vi "io_clear_buffers.vi"(6 "Block Logging (F)":bool, 8 "error in":errorcluster, 11 "VISA resource name":refnum<visa-resource-name>) -> (0 "error out":errorcluster, 3 "VISA resource name out":refnum<visa-resource-name>)   [LabVIEW 2014, in "rszvl_rsidr_core.lvlib"]
uses:
  rszvl_rsidr_core.lvlib
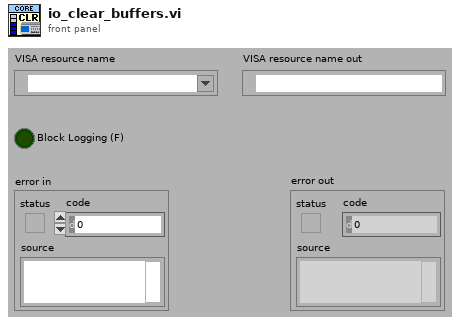
[diagram p1: front panel]
types:
  T1 = typedef "rszvl_rsidr_core.lvlib/type_Session_Data.ctl" = cluster{"Instr type":string, "Instr type for err. msg.":string, "Installed Options":string[], "OPC Timeout":i32, "Query Instrument Status":bool, "Check Range":bool, "Check Options":bool, "Add LF to Write":bool, "Simulate":bool, "Logging":bool, "Logging params":variant, "Interface Type":enum16{"Unknown", "GPIB", "VXI", "GPIB_VXI", "ASRL", "PXI", "TCPIP", "USB", "SOCKET"}, "Fast Sweep":i32, "AdditionalFlags":i32, "WaitBeforeWrite":i32, "WaitBeforeRead":i32, "BinDataChunkSize":i64}
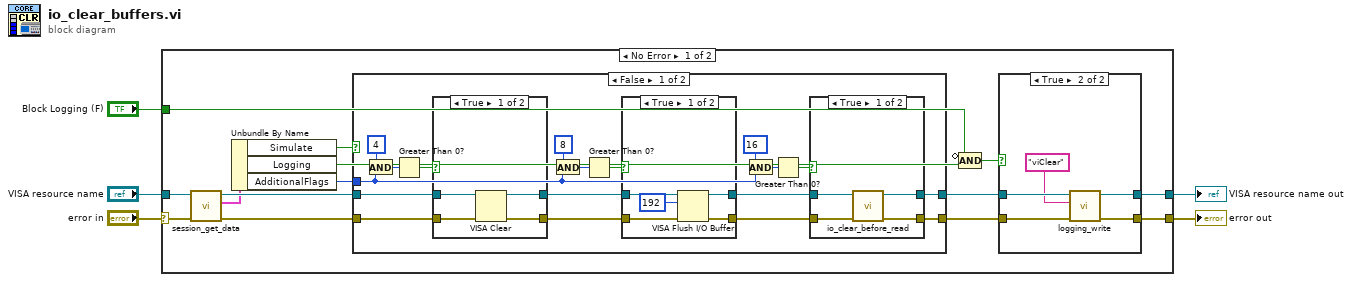
[diagram p0: block diagram]
diagram:
  n1 = case shown="No Error" "error in" {
    selector: "error in" -> [w19 w67]
    tunnel: [w13 w67] -> w1
    tunnel: "VISA resource name" -> [w18 w66]
    tunnel: [w10 w66] -> w2
    tunnel: "Block Logging (F)" -> [w6 _]
    frame No Error {
      n2 = call "session_get_data.vi"("error in"=w19, "VISA resource name"=w18) -> ("error out"=w17:errorcluster, "Session User Data out"=w15:T1, "VISA resource name out"=w16:refnum<visa-resource-name>)  [unwired: 7 in]
      n3 = Unbundle By Name(w15) -> ("Simulate"=w14:bool, "Logging"=w9:bool, "AdditionalFlags"=w7:i32)
      n4 = case shown="False" w14 {
        tunnel: [w37 w65] -> w12
        tunnel: w17 -> [w44 w65]
        tunnel: w16 -> [w43 w64]
        tunnel: [w36 w64] -> w11
        tunnel: w7 -> [w28 _]
        frame False {
          n5 = And(x=4, y=w28) -> (x .and. y?=w41:i32)
          n6 = Greater Than 0?(x=w41) -> (x > 0?=w40:bool)
          n7 = case shown="True" w40 {
            tunnel: w44 -> [w61 w62]
            tunnel: w43 -> [w60 w63]
            tunnel: [w59 w62] -> w39
            tunnel: [w58 w63] -> w38
            frame True {
              n8 = VISA Clear(VISA resource name=w60, error in (no error)=w61) -> (VISA resource name out=w58:refnum<visa-resource-name>, error out=w59:errorcluster)
            }
            frame False {
            }
          }
          n9 = And(x=8, y=w28) -> (x .and. y?=w33:i32)
          n10 = Greater Than 0?(x=w33) -> (x > 0?=w31:bool)
          n11 = case shown="True" w31 {
            tunnel: w39 -> [w54 w57]
            tunnel: w38 -> [w53 w56]
            tunnel: [w52 w57] -> w35
            tunnel: [w51 w56] -> w34
            frame True {
              n12 = VISA Flush I/O Buffer(VISA resource name=w53, mask (16)=u16 192, error in (no error)=w54) -> (VISA resource name out=w51:refnum<visa-resource-name>, error out=w52:errorcluster)
            }
            frame False {
            }
          }
          n13 = And(x=16, y=w28) -> (x .and. y?=w29:i32)
          n14 = Greater Than 0?(x=w29) -> (x > 0?=w27:bool)
          n15 = case shown="True" w27 {
            tunnel: w35 -> [w48 w50]
            tunnel: w34 -> [w47 w49]
            tunnel: [w46 w50] -> w37
            tunnel: [w45 w49] -> w36
            frame True {
              n16 = call "io_clear_before_read.vi"("error in"=w48, "VISA resource name"=w47) -> ("error out"=w46:errorcluster, "VISA resource name out"=w45:refnum<visa-resource-name>)  [unwired: 8 in]
            }
            frame False {
            }
          }
        }
        frame True {
        }
      }
      n17 = Compound Arithmetic op=AND(invert w6, w9) -> (w8:bool)
      n18 = case shown="True" w8 {
        tunnel: w12 -> [w21 w26]
        tunnel: [w21 w24] -> w13
        tunnel: w11 -> [w20 w25]
        tunnel: [w20 w23] -> w10
        frame False {
        }
        frame True {
          n19 = call "logging_write.vi"("error in"=w26, "String to write"="viClear", "VISA resource name"=w25) -> ("error out"=w24:errorcluster, "VISA resource name out"=w23:refnum<visa-resource-name>)  [unwired: 7 in]
        }
      }
    }
    frame Error {
    }
  }
  "VISA resource name out" <- w2
  "error out" <- w1
